vi "CalcDist3D.vi"(9 "element 2":cluster{"X":dbl, "Y":dbl, "Z":dbl}, 10 "element 1":cluster{"X":dbl, "Y":dbl, "Z":dbl}) -> (2 "Distance":dbl)   [LabVIEW 2014]
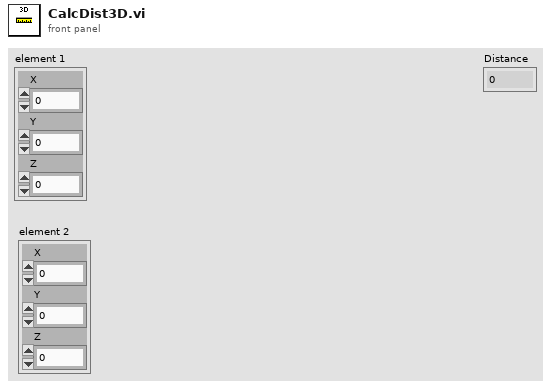
[diagram p1: front panel]
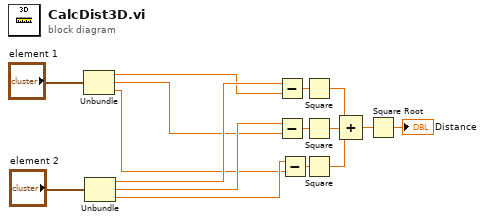
[diagram p0: block diagram]
diagram:
  n1 = Unbundle("element 1") -> ("X"=w10:dbl, "Y"=w8:dbl, "Z"=w5:dbl)
  n2 = Unbundle("element 2") -> ("X"=w11:dbl, "Y"=w9:dbl, "Z"=w6:dbl)
  n3 = Subtract(x=w11, y=w10) -> (x-y=w16:dbl)
  n4 = Subtract(x=w9, y=w8) -> (x-y=w15:dbl)
  n5 = Subtract(x=w6, y=w5) -> (x-y=w7:dbl)
  n6 = Square(x=w16) -> (x^2=w4:dbl)
  n7 = Square(x=w15) -> (x^2=w3:dbl)
  n8 = Square(x=w7) -> (x^2=w2:dbl)
  n9 = Compound Arithmetic op=ADD(w4, w3, w2) -> (w1:dbl)
  n10 = Square Root(x=w1) -> (sqrt(x)=→"Distance":dbl)
